vi "Register Test.vi"(6 "Call Chain":string[](array[string]), 8 "error in (no error)":errorcluster, 10 "Name":string, 11 "Test Manager in":refnum<class "Test Manager.lvclass">) -> (0 "error out":errorcluster, 3 "Test Manager out":refnum<class "Test Manager.lvclass">)   [LabVIEW 2009, in "Caraya.lvlib" / "Test Manager.lvclass"]
uses:
  Test Manager.lvclass
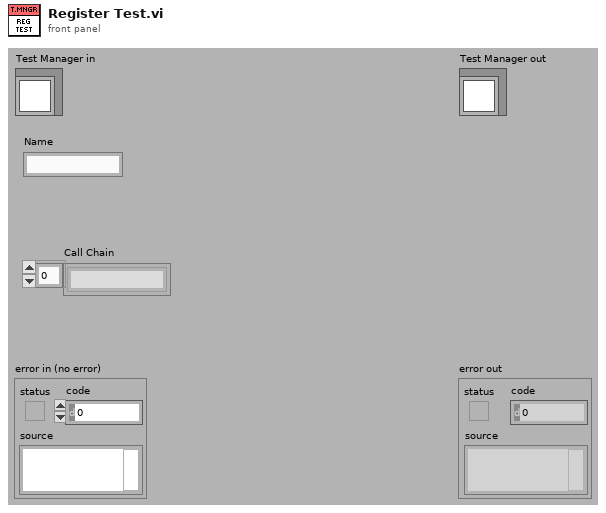
[diagram p1: front panel]
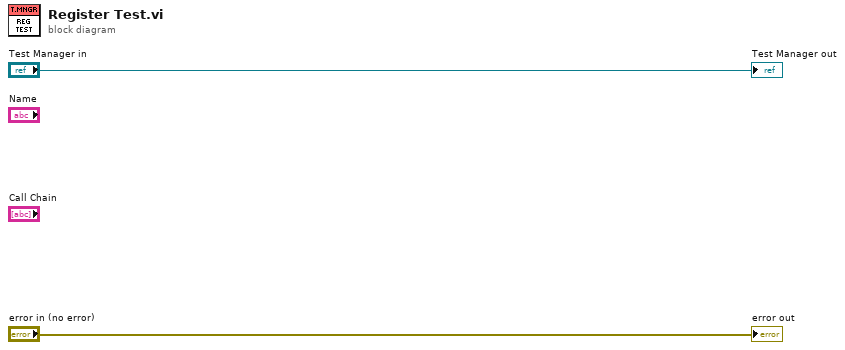
[diagram p0: block diagram]
diagram:
  "error out" <- "error in (no error)"
  "Test Manager out" <- "Test Manager in"
